vi "set_shutter.vi"(8 "error in (no error)":errorcluster, 10 "GenericShutter.lvclass":refnum<class "GenericShutter.lvclass">=refnum, 11 "ScanHeadMH100729FPGA in":refnum<class "ScanHeadMH100729FPGA.lvclass">) -> (0 "error out":errorcluster, 3 "ScanHeadMH100729FPGA out":refnum<class "ScanHeadMH100729FPGA.lvclass">)   [LabVIEW 2010]
uses:
  ScanHeadMH100729FPGA.lvclass
  Shutter/GenericShutter/GenericShutter/GenericShutter.lvclass
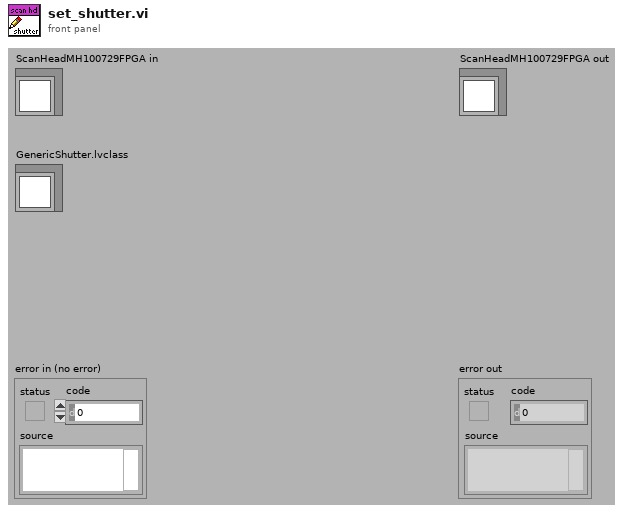
[diagram p1: front panel]
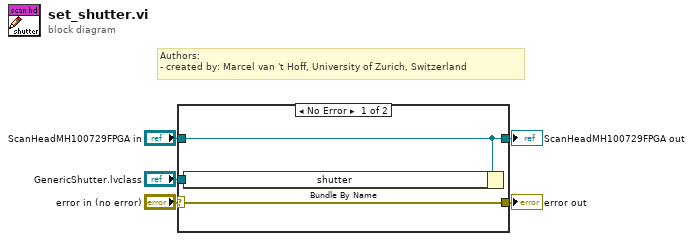
[diagram p0: block diagram]
diagram:
  # "Authors: \n- created by: Marcel van 't Hoff, University of Zurich, Switzerland"
  n1 = case shown="No Error" "error in (no error)" {
    selector: "error in (no error)" -> [w8 w10]
    tunnel: [w8 w10] -> w4
    tunnel: [w7 w9] -> w2
    tunnel: "ScanHeadMH100729FPGA in" -> [w7 w9]
    tunnel: "GenericShutter.lvclass" -> [w6 _]
    frame No Error {
      n2 = Bundle By Name(cluster=w7, "shutter"=w6) -> ()  [unwired: 1 out]
    }
    frame Error {
    }
  }
  "error out" <- w4
  "ScanHeadMH100729FPGA out" <- w2
